vi "EndInterTrial.vi"(8 "error in (no error)":errorcluster, 11 "TrialBasedExperiment in":refnum<class "MatlabExperiment.lvclass">) -> (0 "error out":errorcluster, 3 "TrialBasedExperiment out":refnum<class "MatlabExperiment.lvclass">)   [LabVIEW 2010, in "MatlabExperiment.lvclass"]
uses:
  MatlabExperiment.lvclass
  TrialBasedExperimentObject/TrialBasedExperiment.lvclass
  Matlab API/Matlab API.lvlib
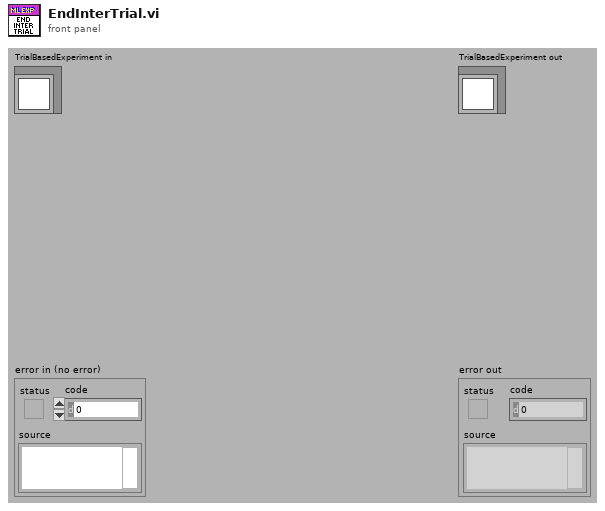
[diagram p1: front panel]
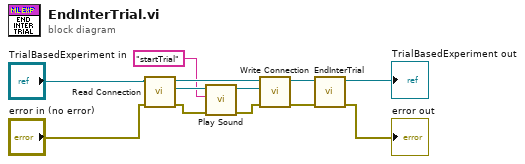
[diagram p0: block diagram]
diagram:
  n1 = call-dynamic "Read Connection.vi"("error in (no error)"="error in (no error)", "TrialBasedExperiment in"="TrialBasedExperiment in") -> ("error out"=w6:errorcluster, "Connection"=w10:refnum<k5>, "TrialBasedExperiment out"=w11:refnum<class "MatlabExperiment.lvclass">)  [unwired: 7 in]
  n2 = call "Play Sound.vi"("error in (no error)"=w6, "Sound Type"="startTrial", "Matlab Connection"=w10) -> ("error out"=w5:errorcluster, "connection ID out"=w9:refnum<k5>)  [unwired: 7 out]
  n3 = call-dynamic "Write Connection.vi"("error in (no error)"=w5, "Connection"=w9, "TrialBasedExperiment in"=w11) -> ("error out"=w4:errorcluster, "TrialBasedExperiment out"=w3:refnum<class "MatlabExperiment.lvclass">)  [unwired: 7 in]
  n4 = call-parent "EndInterTrial.vi"("error in (no error)"=w4, "TrialBasedExperiment in"=w3) -> ("error out"=→"error out":errorcluster, "TrialBasedExperiment out"=→"TrialBasedExperiment out":refnum<class "MatlabExperiment.lvclass">)  [unwired: 8 in]
